vi "Run.vi"(7 "Team Index":i32, 8 "Column":i32, 9 "Row":i32, 10 "View":i32[](array[numeric]) caption="View (Team Index, -1: empty)", 11 "Random In":refnum<class "Random.lvclass">) -> (0 "Replicated":refnum<class "Square.lvclass">, 1 "Direction":T1, 2 "Action":T2, 3 "Random Out":refnum<class "Random.lvclass">)   [LabVIEW 2015, in "Random.lvclass"]
uses:
  Random.lvclass
  Type Defs/Action Enum.ctl
  Type Defs/Direction Enum.ctl
  Square/Square.lvclass
  SubVIs/Read-Only Globals.vi
  SubVIs/Globals (private).vi
  Type Defs/SB Type Defs.lvlib
panel:
  # "NW\nN\nNE\nE\nSE\nS\nSW\nW"
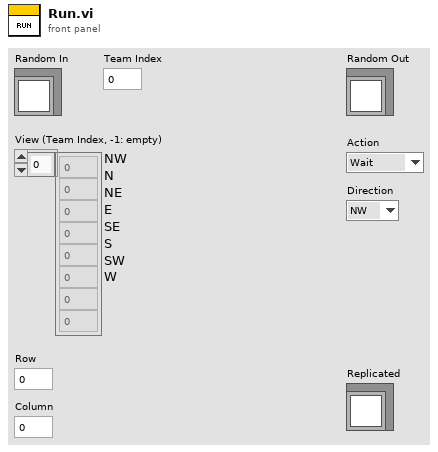
[diagram p1: front panel]
types:
  T1 = typedef "SB Type Defs.lvlib/Direction Enum.ctl" = enum16{"NW", "N", "NE", "E", "SE", "S", "SW", "W"}
  T2 = typedef "SB Type Defs.lvlib/Action Enum.ctl" = enum16{"Wait", "Move", "Attack", "Replicate"}
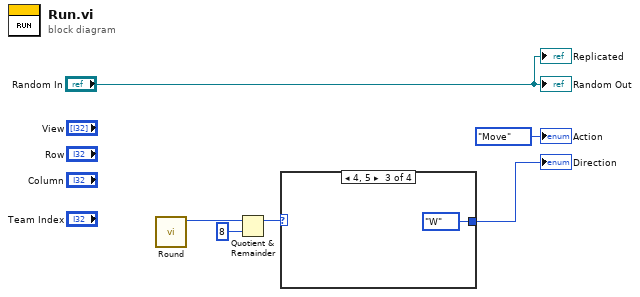
[diagram p0: block diagram]
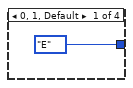
[diagram p2: hidden frame]
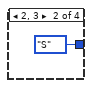
[diagram p3: hidden frame]
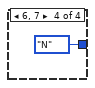
[diagram p4: hidden frame]
diagram:
  n1 = call "Round.vi"() -> ("Round"=w5:i32)  [unwired: 11 in]
  n2 = Quotient & Remainder(x=w5, y=8) -> (x-y*floor(x/y)=w2:i32)  [unwired: 1 out]
  n3 = case shown="4, 5" w2 {
    tunnel: [Direction_Enum."E" ("Direction") Direction_Enum."S" ("Direction") Direction_Enum."W" ("Direction") Direction_Enum."N" ("Direction")] -> w1
    frame 0, 1, Default {
    }
    frame 2, 3 {
    }
    frame 4, 5 {
    }
    frame 6, 7 {
    }
  }
  "Direction" <- w1
  "Random Out" <- "Random In"
  "Action" <- Action_Enum."Move" ("Action")
  "Replicated" <- "Random In"
